vi "Destroy.vi"(0 "reference in":refnum<class "BME280.lvclass">, 5 "error in (no error)":errorcluster) -> (14 "reference out":refnum<class "BME280.lvclass">, 19 "error out":errorcluster)   [LabVIEW 2014, in "BME280.lvclass"]
uses:
  BME280.lvclass
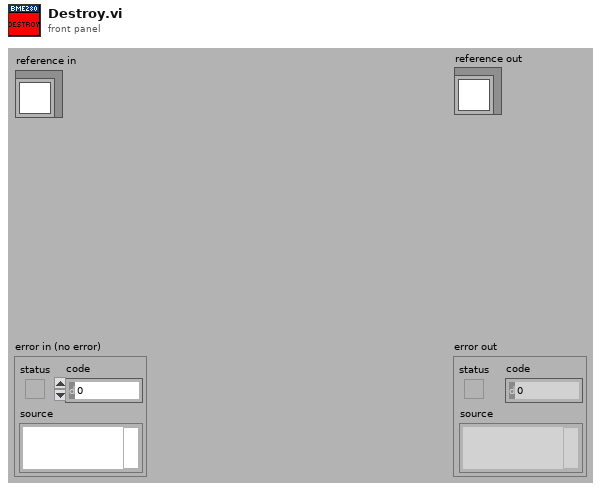
[diagram p1: front panel]
types:
  T1 = typedef "BME280.lvclass/ObjectAttributes.ctl" = cluster{"I2C Slave Address":u8, "TrimmingParameters":T2, "t_fine":i32}
  T2 = typedef "BME280.lvclass/TrimmingParameters.ctl" = cluster{"dig_T1":u16, "dig_T2":i16, "dig_T3":i16, "dig_P1":u16, "dig_P2":i16, "dig_P3":i16, "dig_P4":i16, "dig_P5":i16, "dig_P6":i16, "dig_P7":i16, "dig_P8":i16, "dig_P9":i16, "dig_H1":u8, "dig_H2":i16, "dig_H3":u8, "dig_H4":i16, "dig_H5":i16, "dig_H6":i8}
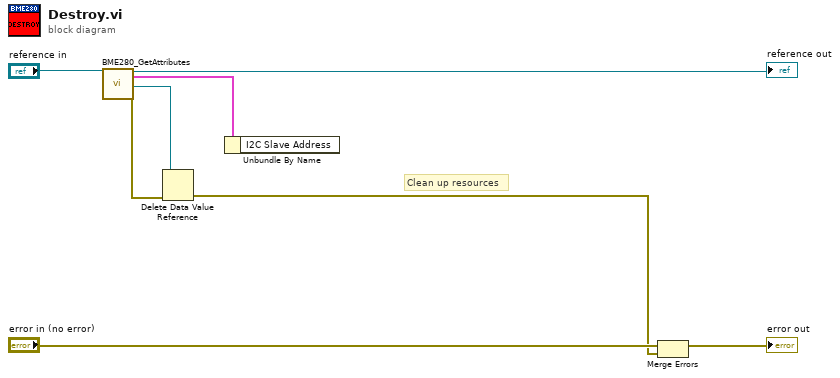
[diagram p0: block diagram]
diagram:
  # "Clean up resources"
  n1 = call "BME280_GetAttributes.vi"("reference in"="reference in") -> ("reference out"=→"reference out":refnum<class "BME280.lvclass">, "Data"=w3:T1, "DataRef"=w4:refnum<data-value>, "error out"=w5:errorcluster)  [unwired: 15 in]
  n2 = Delete Data Value Reference(data value reference=w4, error in=w5) -> (error out=w1:errorcluster)  [unwired: 1 out]
  n3 = Unbundle By Name(w3) -> ()  [unwired: 1 out]
  n4 = Merge Errors("error in (no error)", w1) -> (→"error out":errorcluster)
